vi "VirtualBigAccDAQ.vi"() -> ()   [LabVIEW 2013]
uses:
  <vilib>/Utility/miscctls.llb/LVPointTypeDef.ctl
  Controls/Dust_Event.ctl
  Controls/Signal.ctl
  Controls/Role ID.ctl
  Controls/Hardware ID.ctl
  Controls/Estimate_source.ctl
  <userlib>/_OpenG.lib/numeric/numeric.llb/Random Number Within Range - I32__ogtk.vi
  <userlib>/_OpenG.lib/numeric/numeric.llb/Random Number Within Range - DBL__ogtk.vi
  Global Variables/PSU updated.vi
  <userlib>/_OpenG.lib/comparison/comparison.llb/DBL Changed__ogtk.vi
panel:
  in  "Run":bool
  in  "Filter":bool
  in  "Filter Half Width":i32=10
  out "Random":bool
  in  "User Select":bool
  in  "User Selected Dust ID":i32=2633939
  out "Original Dust ID":i32
  in  "Read new file":bool
  out "Detectors 1 and 2":waveform(dbl)[](graph)
  in  "Write to Database?":bool
  out "PSU":dynamicdata(graph)
  out "Detector 3":dynamicdata(graph)
  out "Avg. Rate":dbl format="%#.3g"
  in  "Reset Count":bool
  in  "min sample rate":dbl=1000000.0 format="%.2p"
  in  "Clear Errors?":bool
  out "No. of Events":i32
  out "error out":errorcluster
  in  "stop":bool
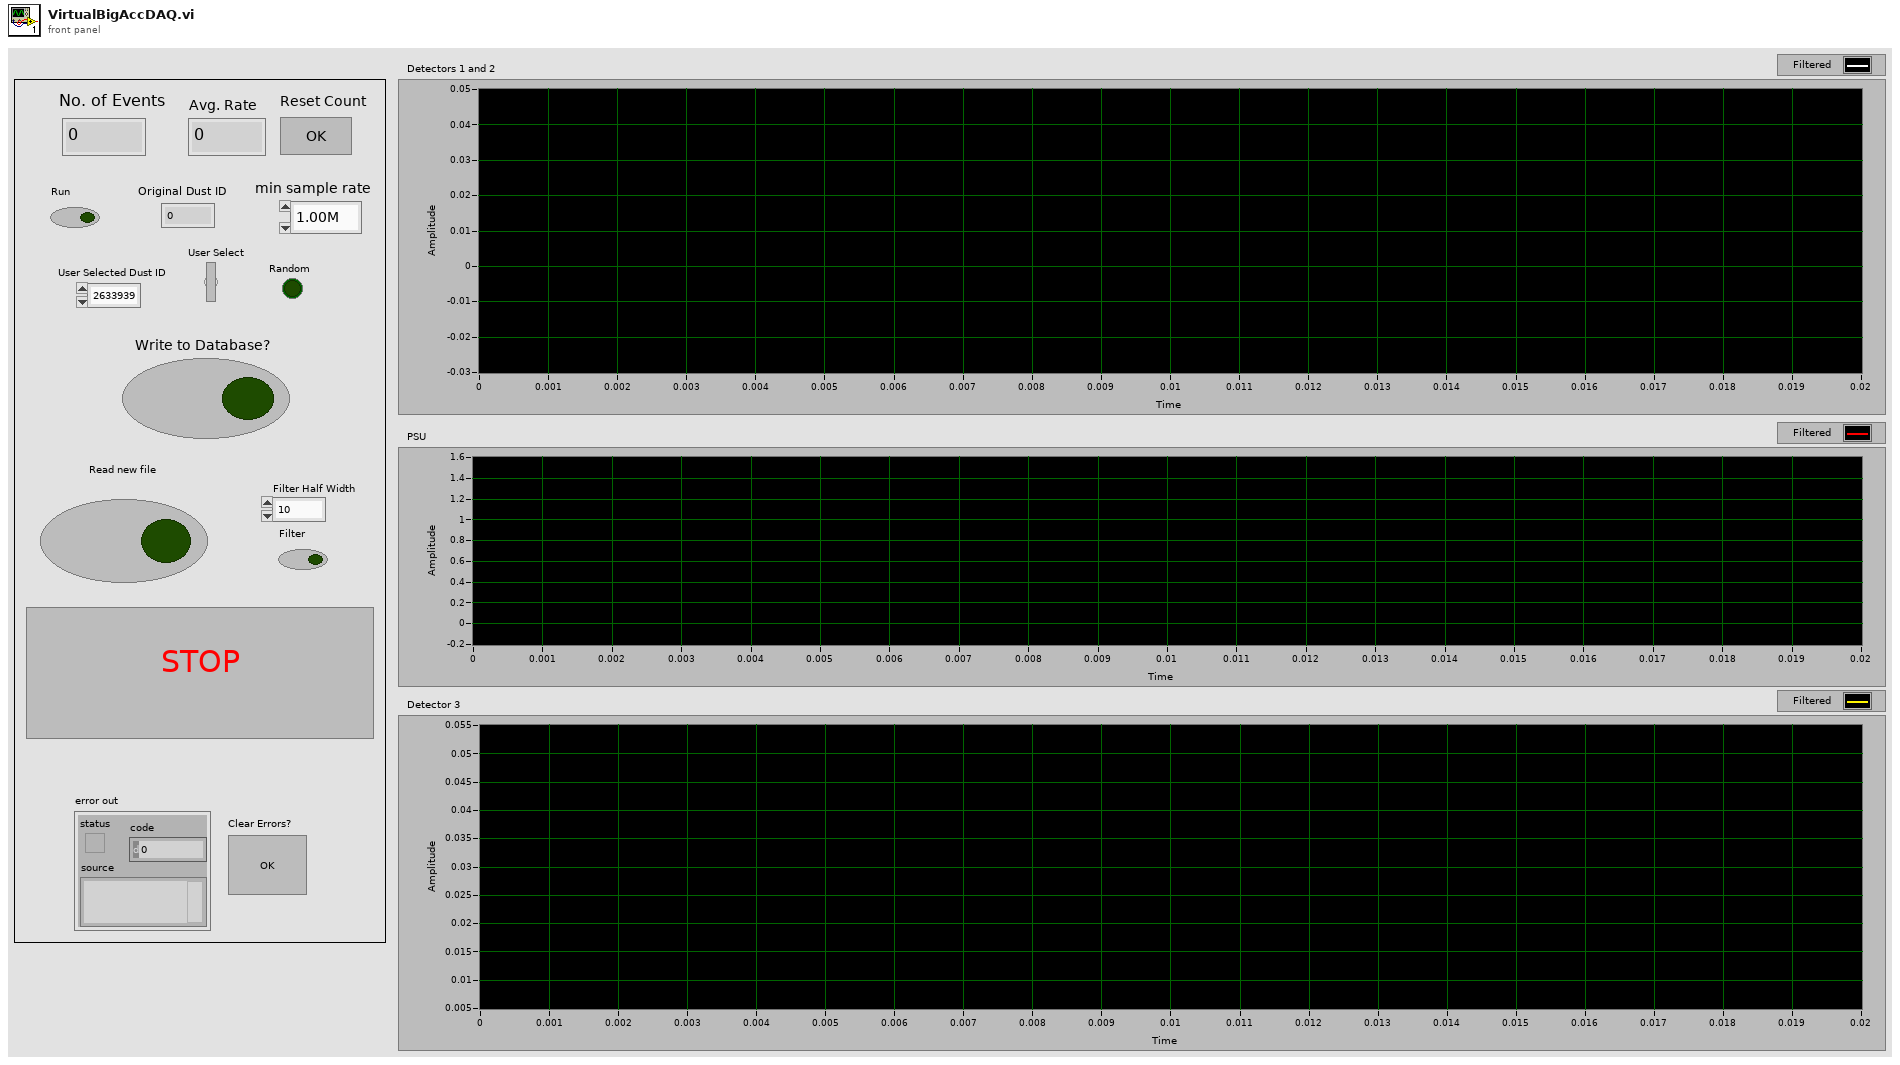
[diagram p1: front panel]
types:
  T1 = typedef "LVPointTypeDef.ctl" = cluster{"Horizontal":i16, "Vertical":i16}
  T2 = cluster{"relativeInitialX":dbl, "xIncrement":dbl, "wfm":dbl[]}
  T3 = typedef "Dust_Event.ctl" = cluster{"Time Stamp":timestamp, "Velocity":sgl, "Mass":sgl, "Charge":sgl, "Radius":sgl, "Array":T4[], "Dust Event ID":i64, "Passed_3rd_Detector":bool, "Estimate Source":T7, "Estimate Quality":sgl}
  T4 = typedef "Signal.ctl" = cluster{"Signal ID":i64, "Time Stamp":timestamp, "Dust Event ID":i64, "Role ID":T5, "Data":sgl[], "Signal Length":i32, "dt":sgl, "Offset":dbl, "Hardware ID":T6}
  T5 = typedef "Role ID.ctl" = enum16{"First_Detector", "Second_Detector", "Third_Detector", "LeCroy_CH1", "LeCroy_CH2", "LeCroy_CH3", "LeCroy_CH4", "PSU", "DCS 1", "DCS 2"}
  T6 = typedef "Hardware ID.ctl" = enum16{"Unknown", "CSA 1", "CSA 2", "CSA 3", "CSA 4", "CSA 5", "CSA 6", "DCS 1", "DCS 2"}
  T7 = typedef "Estimate_source.ctl" = i8
  T8 = typedef "Waveforms.ctl" = cluster{"id_dust_event":u64, "Time Stamp":timestamp, "Velocity":dbl, "Mass":dbl, "Charge":dbl, "Radius":dbl, "Waveform Graph":sgl[][], "Quality":i32}
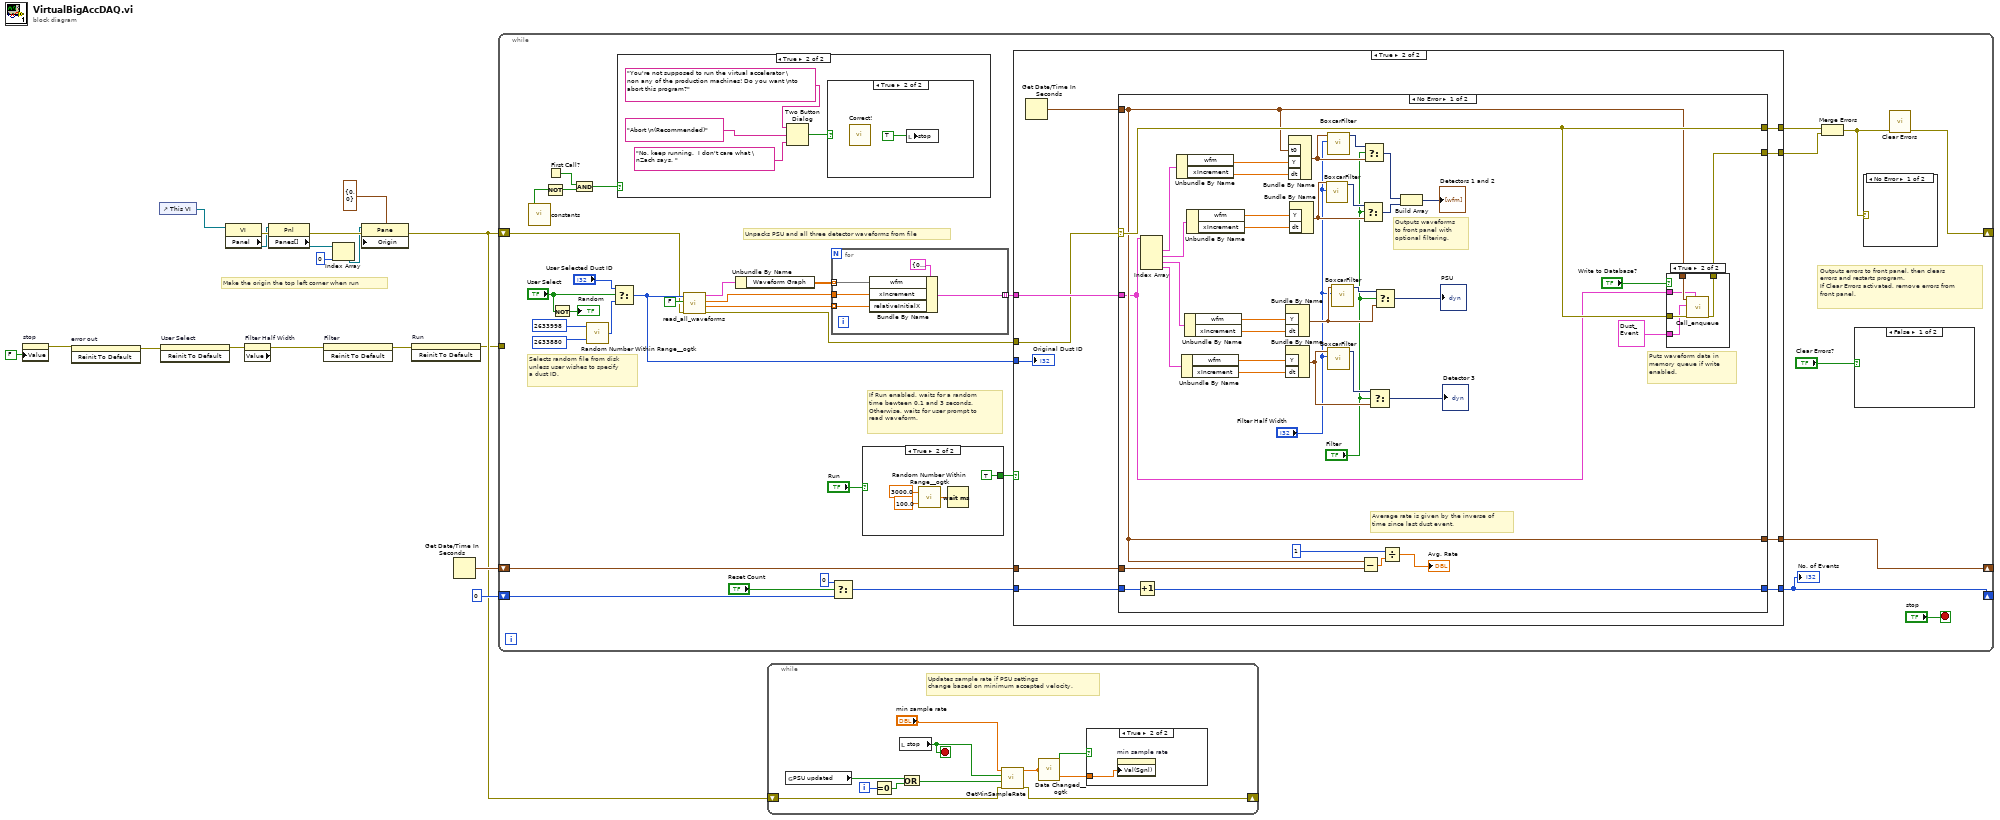
[diagram p0: block diagram]
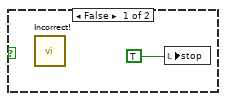
[diagram p4: hidden frame]
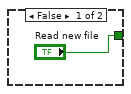
[diagram p5: hidden frame]
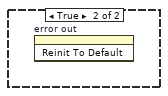
[diagram p9: hidden frame]
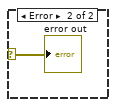
[diagram p10: hidden frame]
diagram:
  # "Make the origin the top left corner when run"
  n1 = property on="stop" class="Bool (strict)"("Value"=FALSE ("stop")) -> (error out=w8:errorcluster)  [unwired: 2 in, 1 out]
  n2 = invoke on="error out" class="Clust (strict)" method="Reinit To Default"(error in=w8) -> (error out=w5:errorcluster)  [unwired: 2 in, 2 out]
  n3 = control-ref of="This VI"() -> (w11:refnum<vi>)
  n4 = invoke on="User Select" class="Bool (strict)" method="Reinit To Default"(error in=w5) -> (error out=w4:errorcluster)  [unwired: 2 in, 2 out]
  n5 = property class="VI"(reference=w11) -> (error out=w18:errorcluster, "Panel"=w12:refnum<vi>)  [unwired: 1 in, 1 out]
  n6 = property on="Filter Half Width" class="DigNum (strict)" props=["Value"](error in=w4) -> (error out=w3:errorcluster)  [unwired: 1 in, 2 out]
  n7 = property class="Pnl"(reference=w12, error in=w18) -> (error out=w17:errorcluster, "Panes[]"=w16:refnum<vi>[])  [unwired: 1 out]
  n8 = invoke on="Filter" class="Bool (strict)" method="Reinit To Default"(error in=w3) -> (error out=w2:errorcluster)  [unwired: 2 in, 2 out]
  n9 = Index Array(array=w16, index=0) -> (element=w14:refnum<vi>)
  n10 = property class="Pane"(reference=w14, error in=w17, "Origin"=T1 {"Horizontal"=0, "Vertical"=0}) -> (error out=w6:errorcluster)  [unwired: 1 out]
  n11 = invoke on="Run" class="Bool (strict)" method="Reinit To Default"(error in=w2) -> (error out=w1:errorcluster)  [unwired: 2 in, 2 out]
  n12 = Get Date/Time In Seconds() -> (seconds since 1Jan1904=w7:timestamp)
  n13 = while {
    shift-right: [w50] -> _
    shift-left: w6 -> [w19]
    shift-right: [w29] -> _
    shift-left: 0 -> [w44]
    shift-right: [w45] -> _
    shift-left: w7 -> [w47]
    tunnel: w1 -> [_]
    stop <- "stop" stop-if-true
    # "If Run enabled, waits for a random\ntime bewteen 0.1 and 3 seconds. \nOtherwise, waits for user prompt to \nread waveform."
    # "Unpacks PSU and all three detector waveforms from file"
    # "Selects random file from disk\nunless user wishes to specify\na dust ID."
    # "Outputs errors to front panel, then clears \nerrors and restarts program. \nIf Clear Errors activated, remove errors from \nfront panel."
    n14 = call "constants.vi"() -> ("Testing"=w20:bool)  [unwired: 3 out]
    n15 = Not(x=w20) -> (.not. x?=w22:bool)
    n16 = First Call?() -> (First Call?: T/F=w23:bool)
    n17 = Not(x="User Select") -> (.not. x?=→"Random":bool)
    n18 = And(x=w23, y=w22) -> (x .and. y?=w21:bool)
    n19 = call-poly <userlib>:"Random Number Within Range__ogtk.vi"("High"=2633998, "Low"=2633880) -> ("Random Number"=w32:i32)  [unwired: 3 in]
    n20 = Select(t="User Selected Dust ID", s="User Select", f=w32) -> (s? t:f=w33:i32)
    n21 = case shown="True" w21 {
      frame False {
      }
      frame True {
        n22 = Two Button Dialog(message="You're not supposed to run the virtual accelerator \non any of the production machines! Do you want \nto abort this program?", 1:"No, keep running.  I don't care what \nZach says. ", 2:"Abort \n(Recommended)") -> (T button?=w53:bool)
        n23 = case shown="True" w53 {
          frame False {
            n24 = call "Incorrect!"() -> ()  [unwired: 18 in, 2 out]
            n25 = local write "stop"(TRUE) -> ()
          }
          frame True {
            n26 = call "Correct!"() -> ()  [unwired: 18 in, 2 out]
            n27 = local write "stop"(TRUE) -> ()
          }
        }
      }
    }
    n28 = call "read_all_waveforms.vi"("error in (no error)"=w19, "Small?"=FALSE, "Dust Event ID"=w33) -> ("error out"=w28:errorcluster, "Offset Array"=w40:dbl[], "dt"=w41:dbl, "Waveform"=w38:T8)  [unwired: 5 in]
    n29 = Unbundle By Name(w38) -> ("Waveform Graph"=w39:sgl[][])
    n30 = for {
      tunnel: w39 -> [w67] mode=indexing
      tunnel: w40 -> [w65] mode=indexing
      tunnel: w41 -> [w66]
      tunnel: [w64] -> w36 mode=indexing
      n31 = Bundle By Name(cluster=T2 {"relativeInitialX"=0.0, "xIncrement"=0.0, "wfm"=[]}, "wfm"=w67, "xIncrement"=w66, "relativeInitialX"=w65) -> (w64:T2)
    }
    n32 = Select(t=0, s="Reset Count", f=w44) -> (s? t:f=w46:i32)
    n33 = case shown="True" "Run" {
      tunnel: ["Read new file" TRUE ("Read new file")] -> w25
      frame False {
      }
      frame True {
        n34 = call-poly <userlib>:"Random Number Within Range__ogtk.vi"("High"=3000.0, "Low"=100.0) -> ("Random Number"=w61:dbl)  [unwired: 3 in]
        n35 = Wait (ms)(milliseconds to wait=w61) -> ()  [unwired: 1 out]
      }
    }
    n36 = case shown="True" w25 {
      tunnel: [w69 w77] -> w43
      tunnel: [w69 w78] -> w42
      tunnel: w47 -> [w70 w81]
      tunnel: w46 -> [w71 w80]
      tunnel: [w71 w79] -> w29
      tunnel: [w70 w76] -> w45
      tunnel: w36 -> [_ w75]
      tunnel: w33 -> [_ w74]
      tunnel: w28 -> [w69 w72]
      frame False {
      }
      frame True {
        n37 = Get Date/Time In Seconds() -> (seconds since 1Jan1904=w73:timestamp)
        n38 = case shown="No Error" w72 {
          selector: w72 -> [w114 w129]
          tunnel: [w116 w129] -> w77
          tunnel: w80 -> [w115 w128]
          tunnel: [w111 w128] -> w79
          tunnel: [w114 w129] -> w78
          tunnel: w81 -> [w102 w127]
          tunnel: [w98 w127] -> w76
          tunnel: w75 -> [w82 _]
          tunnel: w73 -> [w98 _]
          frame No Error {
            # "Puts waveform data in\nmemory queue if write \nenabled."
            # "Outputs waveforms\nto front panel with\noptional filtering."
            # "Average rate is given by the inverse of \ntime since last dust event."
            n39 = Increment(x=w115) -> (x+1=w111:i32)
            n40 = Index Array(array=w82) -> (element #1=w120:T2, element #2=w119:T2, element #3=w113:T2, element #4=w112:T2)  [unwired: 4 in]
            n41 = Unbundle By Name(w120) -> ("wfm"=w109:dbl[], "xIncrement"=w108:dbl)
            n42 = Unbundle By Name(w112) -> ("wfm"=w105:dbl[], "xIncrement"=w104:dbl)
            n43 = Unbundle By Name(w113) -> ("wfm"=w97:dbl[], "xIncrement"=w103:dbl)
            n44 = Unbundle By Name(w119) -> ("wfm"=w107:dbl[], "xIncrement"=w106:dbl)
            n45 = Bundle By Name("Y"=w97, "dt"=w103) -> (w86:waveform(dbl))  [unwired: 1 in]
            n46 = Bundle By Name("Y"=w105, "dt"=w104) -> (w95:waveform(dbl))  [unwired: 1 in]
            n47 = Bundle By Name("t0"=w98, "Y"=w109, "dt"=w108) -> (w89:waveform(dbl))  [unwired: 1 in]
            n48 = Bundle By Name("Y"=w107, "dt"=w106) -> (w91:waveform(dbl))  [unwired: 1 in]
            n49 = call "BoxcarFilter.vi"("Half Width"="Filter Half Width", "Signal"=w91) -> ("Filtered Signal"=w90:dynamicdata)  [unwired: 8 in, 1 out]
            n50 = call "BoxcarFilter.vi"("Half Width"="Filter Half Width", "Signal"=w89) -> ("Filtered Signal"=w93:dynamicdata)  [unwired: 8 in, 1 out]
            n51 = call "BoxcarFilter.vi"("Half Width"="Filter Half Width", "Signal"=w95) -> ("Filtered Signal"=w96:dynamicdata)  [unwired: 8 in, 1 out]
            n52 = call "BoxcarFilter.vi"("Half Width"="Filter Half Width", "Signal"=w86) -> ("Filtered Signal"=w87:dynamicdata)  [unwired: 8 in, 1 out]
            n53 = Subtract(x=w98, y=w102) -> (x-y=w100:dbl)
            n54 = Select(t=w90, s="Filter", f=w91) -> (s? t:f=w92:dynamicdata)
            n55 = Select(t=w93, s="Filter", f=w89) -> (s? t:f=w88:dynamicdata)
            n56 = Select(t=w96, s="Filter", f=w95) -> (s? t:f=→"Detector 3":dynamicdata)
            n57 = Select(t=w87, s="Filter", f=w86) -> (s? t:f=→"PSU":dynamicdata)
            n58 = Divide(x=1 ("y"), y=w100) -> (x/y=→"Avg. Rate":dbl)
            n59 = Build Array(w88, w92) -> (→"Detectors 1 and 2":dynamicdata[])
            n60 = case shown="True" "Write to Database?" {
              tunnel: w114 -> [w121 w126]
              tunnel: [w121 w125] -> w116
              tunnel: T3 {"Time Stamp"=timestamp(0 s since 1904-01-01), "Velocity"=0.0, "Mass"=0.0, "Charge"=0.0, "Radius"=0.0, "Array"=[], "Dust Event ID"=0, "Passed_3rd_Detector"=FALSE, "Estimate Source"=0, "Estimate Quality"=0.0} ("Input Data") -> [_ w124]
              tunnel: w98 -> [_ w123]
              tunnel: w82 -> [_ w122]
              frame False {
              }
              frame True {
                n61 = call "Call_enqueue.vi"("Waveform"=w122, "error in"=w126, "Input Data"=w124, "Timestamp"=w123) -> ("error out"=w125:errorcluster)  [unwired: 7 in]
              }
            }
          }
          frame Error {
          }
        }
        "Original Dust ID" <- w74
      }
    }
    "No. of Events" <- w29
    n62 = Merge Errors(w42, w43) -> (w52:errorcluster)
    n63 = case shown="False" "Clear Errors?" {
      frame False {
      }
      frame True {
        n64 = invoke on="error out" class="Clust (strict)" method="Reinit To Default"() -> ()  [unwired: 3 in, 3 out]
      }
    }
    n65 = case shown="No Error" w52 {
      selector: w52 -> [_ w130]
      frame No Error {
      }
      frame Error {
        "error out" <- w130
      }
    }
    n66 = call <vilib>:"Clear Errors.vi"("error in (no error)"=w52) -> ("error out"=w50:errorcluster)  [unwired: 6 in]
  }
  n67 = while {
    shift-right: [w134] -> _
    shift-left: w6 -> [w137]
    i -> [w140]
    stop <- w135 stop-if-true
    # "Updates sample rate if PSU settings \nchange based on minimum accepted velocity."
    n68 = global read "PSU updated.vi" "PSU updated"() -> (w139:bool)
    n69 = Equal To 0?(x=w140) -> (x = 0?=w138:bool)
    n70 = local read "stop"() -> (w135:bool)
    n71 = Or(x=w139, y=w138) -> (x .or. y?=w136:bool)
    n72 = call "GetMinSampleRate.vi"("error in (no error)"=w137, "PSU Update"=w136, "stop"=w135, "min sample rate"="min sample rate") -> ("error out"=w134:errorcluster, "min sample rate"=w132:dbl)  [unwired: 6 in]
    n73 = call-poly <userlib>:"Data Changed__ogtk.vi"("DBL"=w132) -> ("Changed"=w133:bool)
    n74 = case shown="True" w133 {
      tunnel: w132 -> [_ w141]
      frame False {
      }
      frame True {
        n75 = property on="min sample rate" class="DigNum (strict)"("Val(Sgnl)"=w141) -> ()  [unwired: 2 in, 2 out]
      }
    }
  }
